vi "wyswietlInfoOZrealizowanychPunktach.vi"(4 "Pozostalo punktow":i32, 5 "Rodzaj pomiarow":T1) -> (2 "Zrealizowane punkty info":string)   [LabVIEW 2014]
uses:
  glownaMaszynaStanowVIs/wczytajListePunktowVIs/RodzajPomiarow.ctl
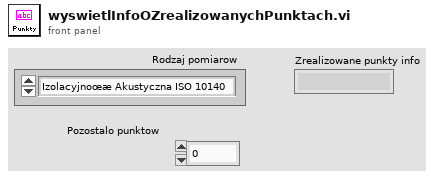
[diagram p1: front panel]
types:
  T1 = typedef "RodzajPomiarow.ctl" = enum16{"Izolacyjnoœæ Akustyczna ISO 10140", "Sekwencja testowa"}
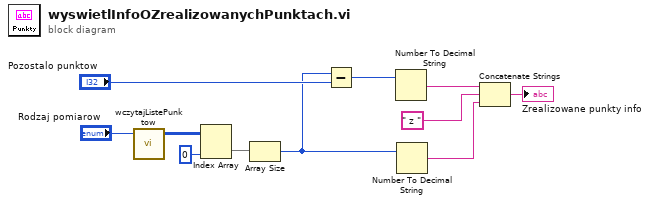
[diagram p0: block diagram]
diagram:
  n1 = call "wczytajListePunktow.vi"("Rodzaj pomiarow"="Rodzaj pomiarow") -> ("Wspolrzedne katowe"=w5:i32[][])  [unwired: 4 in]
  n2 = Index Array(array=w5, index (col)=0 ("disabled index (col)")) -> (element=w3:i32[])  [unwired: 1 in]
  n3 = Array Size(array=w3) -> (size(s)=w1:i32)
  n4 = Subtract(x=w1, y="Pozostalo punktow") -> (x-y=w2:i32)
  n5 = Number To Decimal String(number=w2) -> (decimal integer string=w11:string)  [unwired: 1 in]
  n6 = Number To Decimal String(number=w1) -> (decimal integer string=w10:string)  [unwired: 1 in]
  n7 = Concatenate Strings(w11, " z " ("string"), w10) -> (→"Zrealizowane punkty info":string)
